vi "Stream Arc (FW7).vi"(4 "Direction (0: clockwise)":u16(ring) items=["clockwise", "counter-clockwise"], 5 "End Point":i64[](array[numeric]), 6 "Position Mode (0: absolute)":u16(ring) items=["absolute", "relative"], 7 "Center Point":i64[](array[numeric]), 8 "error in (no error)":errorcluster, 9 "Device Number":string, 10 "Stream Number (1)":u8=1, 11 "VISA resource name":refnum<visa-resource-name>) -> (0 "error out":errorcluster, 3 "VISA resource name out":refnum<visa-resource-name>)   [LabVIEW 2018, in "Zaber A Series.lvlib"]
doc: "Adds a circular arc command to an open stream. The position where the previous stream command leaves the device will be the starting point for the arc. The Center Position input specifies where the center of the circle will be, and the End Point input specified the end of the arc. There is also a Direction input to control which way around the circle the arc is drawn.\n\nThe Position Mode input controls whether the center and endpoint positions are absolute or relative to the arc start.\n\nThe center and end points are specified in microstep units - use the Convert Position to Device Units VI to convert from standard measurements.\n\nThis VI does not check in advance for error conditions such as streams not being supported or the stream not being open.\n\nThis VI requires that the Initialize VI has been called with the same serial port and that the specified stream is open."
uses:
  Zaber A Series.lvlib
  Private/All Commands.ctl
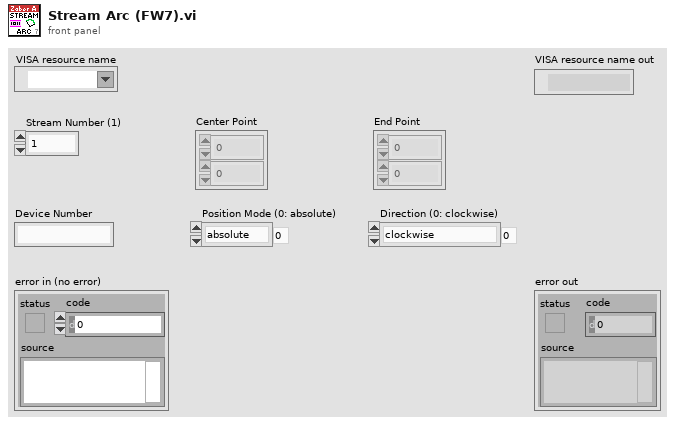
[diagram p1: front panel]
types:
  T1 = typedef "Zaber A Series.lvlib/All Commands.ctl" = string
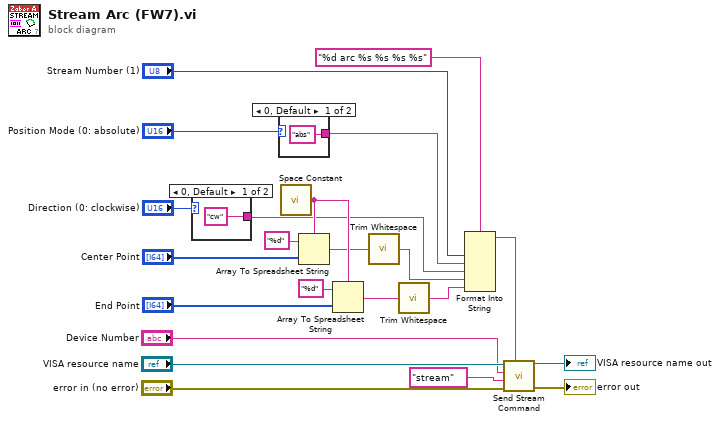
[diagram p0: block diagram]
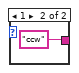
[diagram p2: hidden frame]
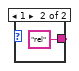
[diagram p3: hidden frame]
diagram:
  n1 = case shown="0, Default" "Direction (0: clockwise)" {
    tunnel: ["cw" "ccw"] -> w6
    frame 0, Default {
    }
    frame 1 {
    }
  }
  n2 = case shown="0, Default" "Position Mode (0: absolute)" {
    tunnel: ["abs" "rel"] -> w7
    frame 0, Default {
    }
    frame 1 {
    }
  }
  n3 = call <vilib>:"Space Constant.vi"() -> ("String"=w12:string)
  n4 = Array To Spreadsheet String(delimiter (Tab)=w12, array="Center Point", 3:"%d" ("format string")) -> (spreadsheet string=w11:string)
  n5 = Array To Spreadsheet String(delimiter (Tab)=w12, array="End Point", 3:"%d" ("format string")) -> (spreadsheet string=w10:string)
  n6 = call <vilib>:"Trim Whitespace.vi"("string"=w11) -> ("trimmed string"=w5:string)  [unwired: 1 in]
  n7 = call <vilib>:"Trim Whitespace.vi"("string"=w10) -> ("trimmed string"=w4:string)  [unwired: 1 in]
  n8 = Format Into String(format string="%d arc %s %s %s %s", "Stream Number (1)", w7, w6, w5, w4) -> (resulting string=w3:string)  [unwired: 2 in, 1 out]
  n9 = call "Send Stream Command.vi"("Data"=w3, "error in (no error)"="error in (no error)", "Command"=T1 "stream" ("Complete Command List"), "Device Number"="Device Number", "VISA resource name"="VISA resource name") -> ("error out"=→"error out":errorcluster, "VISA resource name out"=→"VISA resource name out":refnum<visa-resource-name>)  [unwired: 5 in]
